vi "SAC-Options Dialog.vi"(0 "Options in":T1) -> (4 "Options out":T1, 8 "Canceled?":bool)   [LabVIEW 2020]
uses:
  Typedefs/SAC-Options.ctl
panel:
  in  "Wait (s)":dbl caption="Wait between measurements (s)"
  out "exit signal":bool
  in  "Cancel":bool
  in  "OK":bool
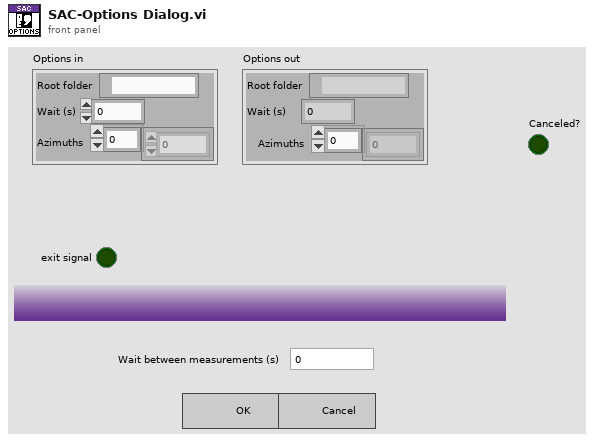
[diagram p1: front panel]
types:
  T1 = typedef "SAC-Options.ctl" = cluster{"Root folder":path, "Wait (s)":dbl, "Azimuths":dbl[]}
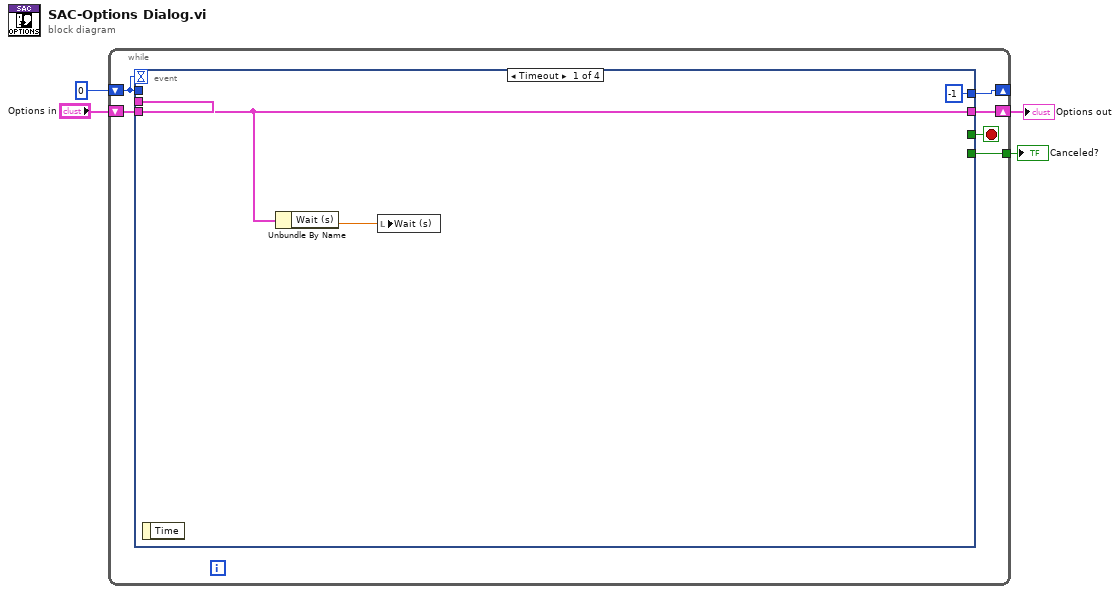
[diagram p0: block diagram]
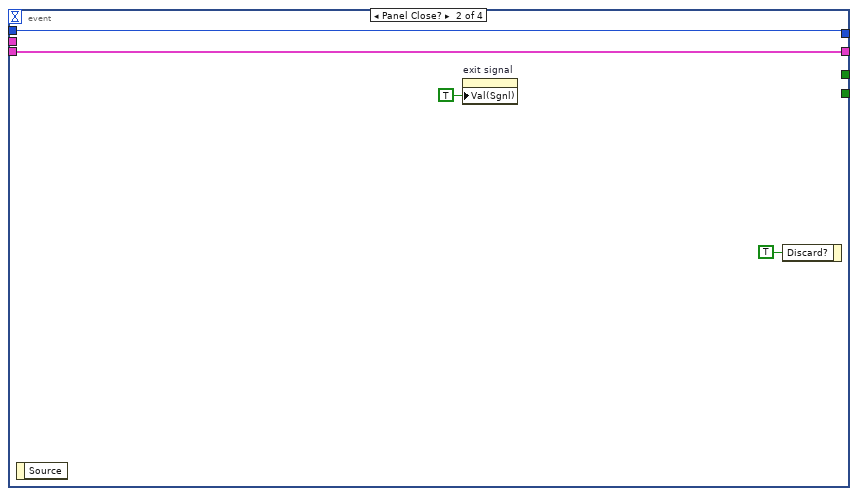
[diagram p2: hidden frame]
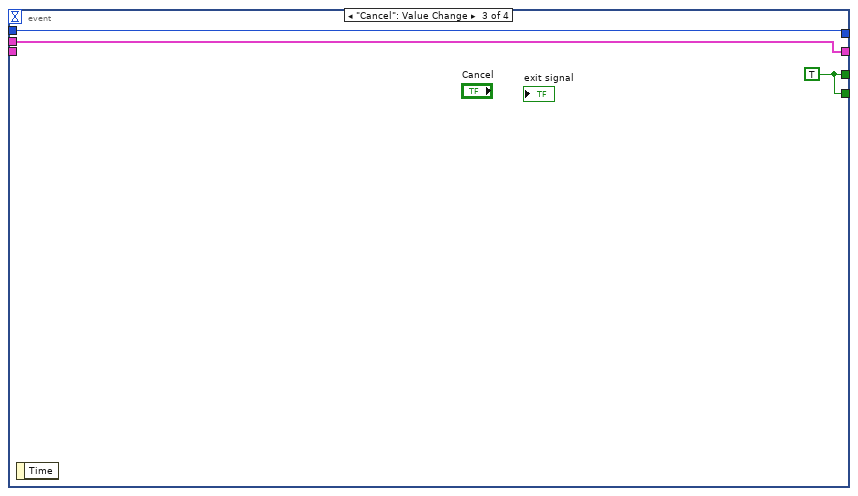
[diagram p3: hidden frame]
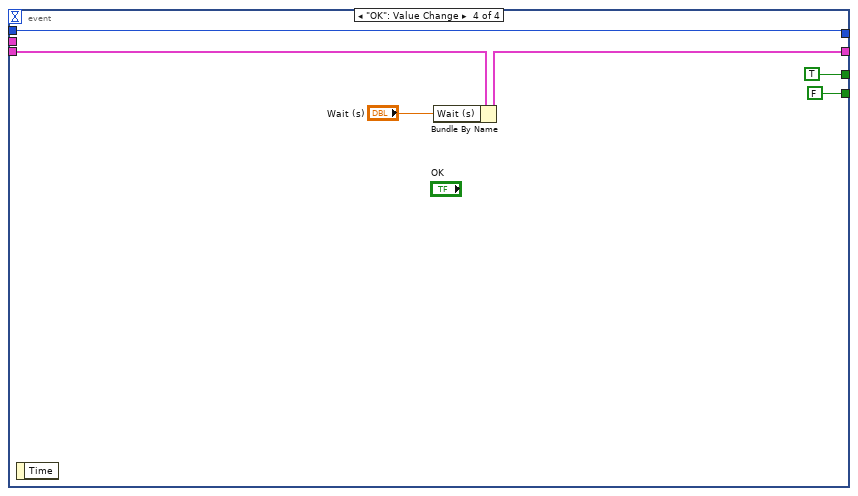
[diagram p4: hidden frame]
diagram:
  n1 = while {
    shift-right: [w10] -> _
    shift-left: 0 -> [w5]
    tunnel: [w7] -> w1
    shift-right: [w9] -> w2
    shift-left: "Options in" -> [w6]
    stop <- w8 stop-if-true
    n2 = event shown="[0] Timeout" {
      selector: _ -> [_ _ _ _]
      dyn-events: _ -> [_ _ _ _]
      timeout: w5 -> [_ _ _ _]
      tunnel: [-1 w17 w18 w23] -> w10
      tunnel: w6 -> [w12 w16 _ w26]
      tunnel: [w12 w16 w19 w22] -> w9
      tunnel: [_ _ w20 TRUE] -> w8
      tunnel: [_ _ w20 FALSE] -> w7
      tunnel: w6 -> [_ _ w19 _]
      tunnel: w5 -> [_ w17 w18 w23]
      event Timeout {
        n3 = event-data() -> ()  [unwired: 1 in, 1 out]
        n4 = Unbundle By Name(w12) -> ("Wait (s)"=w11:dbl)
        n5 = local write "Wait (s)"(w11) -> ()
      }
      event Panel Close? {
        n6 = event-data() -> ()  [unwired: 1 in, 1 out]
        n7 = property on="exit signal" class="Bool (strict)"("Val(Sgnl)"=TRUE ("Value (Signaling)")) -> ()  [unwired: 2 in, 2 out]
        n8 = event-data("Discard?"=TRUE) -> ()  [unwired: 1 in, 1 out]
      }
      event "Cancel": Value Change {
        w20 = TRUE
        n9 = event-data() -> ()  [unwired: 1 in, 1 out]
      }
      event "OK": Value Change {
        n10 = event-data() -> ()  [unwired: 1 in, 1 out]
        n11 = Bundle By Name(cluster=w26, "Wait (s)"="Wait (s)") -> (w22:T1)
      }
    }
  }
  "Options out" <- w2
  "Canceled?" <- w1
